vi "Regular Color Style.vi"(11 "Color Ramp Cluster in":T1={"Color Ramp Style"=enum."None", "Color Ramp Array"=[16711934, 393471, 57855, 4390754, 16449346, 16744722, 16711680], "Color Ramp Index"=[45, 91, 133, 175, 219, 255], "Interpolate?"=FALSE, "Logarithm?"=FALSE}) -> (3 "Color Ramp Cluster out":T1={"Color Ramp Style"=enum."None", "Color Ramp Array"=[16711934, 393471, 57855, 4390754, 16449346, 16744722, 16711680], "Color Ramp Index"=[45, 91, 133, 175, 219, 255], "Interpolate?"=FALSE, "Logarithm?"=FALSE})   [LabVIEW 2020, in "3D Plot.lvclass"]
uses:
  3D Plot.lvclass
  Color Ramp Cluster.ctl
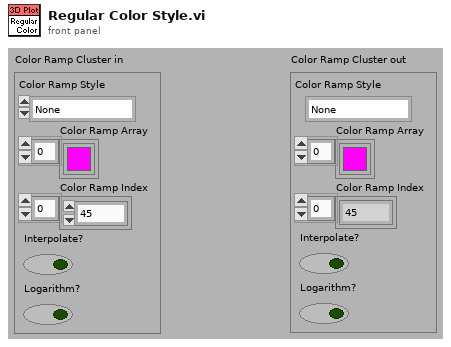
[diagram p1: front panel]
types:
  T1 = typedef "3D Plot.lvclass/Color Ramp Cluster.ctl" = cluster{"Color Ramp Style":enum16{"None", "Shaded", "Color spectrum", "Grey scale", "Custom"}, "Color Ramp Array":u32[], "Color Ramp Index":i32[], "Interpolate?":bool, "Logarithm?":bool}
  T2 = enum16{"None", "Shaded", "Color spectrum", "Grey scale", "Custom"}
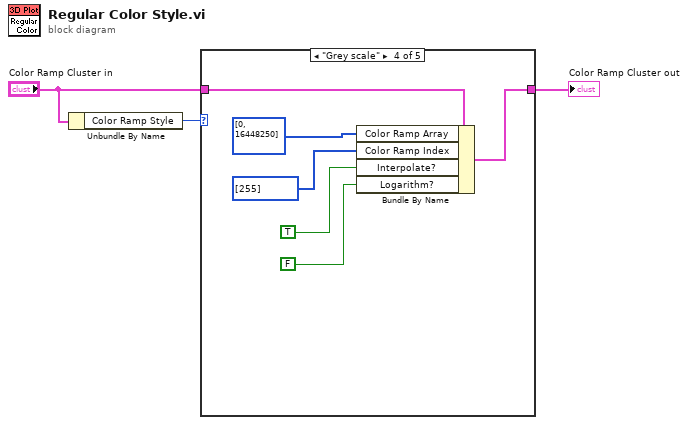
[diagram p0: block diagram]
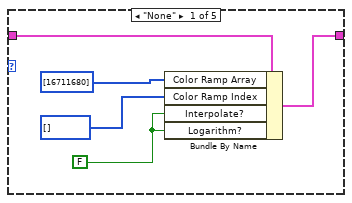
[diagram p2: hidden frame]
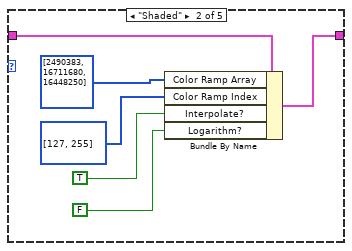
[diagram p3: hidden frame]
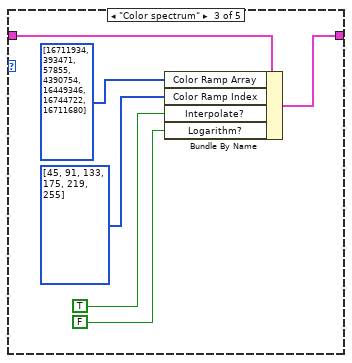
[diagram p4: hidden frame]
diagram:
  n1 = Unbundle By Name("Color Ramp Cluster in") -> ("Color Ramp Style"=w3:T2)
  n2 = case shown="\"Grey scale\"" w3 {
    tunnel: [w5 w10 w15 w21 w27] -> w2
    tunnel: "Color Ramp Cluster in" -> [w8 w11 w16 w22 w27]
    frame "None" {
      w6 = FALSE ("Interpolate?")
      n3 = Bundle By Name(cluster=w8, "Color Ramp Array"=u32[] [16711680], "Color Ramp Index"=u32[] [], "Interpolate?"=w6, "Logarithm?"=w6) -> (w5:T1)
    }
    frame "Shaded" {
      n4 = Bundle By Name(cluster=w11, "Color Ramp Array"=u32[] [2490383, 16711680, 16448250], "Color Ramp Index"=u32[] [127, 255], "Interpolate?"=TRUE, "Logarithm?"=FALSE) -> (w10:T1)
    }
    frame "Color spectrum" {
      n5 = Bundle By Name(cluster=w16, "Color Ramp Array"=u32[] [16711934, 393471, 57855, 4390754, 16449346, 16744722, 16711680], "Color Ramp Index"=i32[] [45, 91, 133, 175, 219, 255], "Interpolate?"=TRUE, "Logarithm?"=FALSE) -> (w15:T1)
    }
    frame "Grey scale" {
      n6 = Bundle By Name(cluster=w22, "Color Ramp Array"=u32[] [0, 16448250], "Color Ramp Index"=u32[] [255], "Interpolate?"=TRUE, "Logarithm?"=FALSE) -> (w21:T1)
    }
    frame "Custom" {
    }
  }
  "Color Ramp Cluster out" <- w2
